vi "prototype-02.vi"() -> ()   [LabVIEW 2026]
uses:
  <vilib>/Instr/_visa.llb/VISA Configure Serial Port (Instr).vi
panel:
  in  "Numeric 3":dbl
  in  "Numeric 2":dbl
  in  "Numeric":dbl
  in  "TV":bool
  in  "BULB":bool
  in  "FAN":bool
  in  "VISA resource name":refnum<visa-resource-name>
  in  "stop":bool
  in  "Voltage":dbl(knob) scale=0.0..250.0
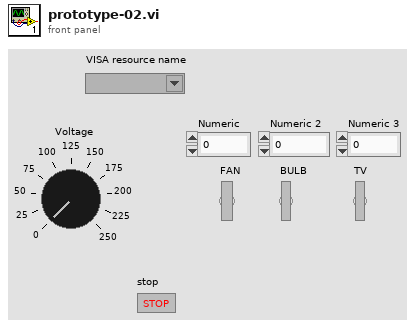
[diagram p1: front panel]
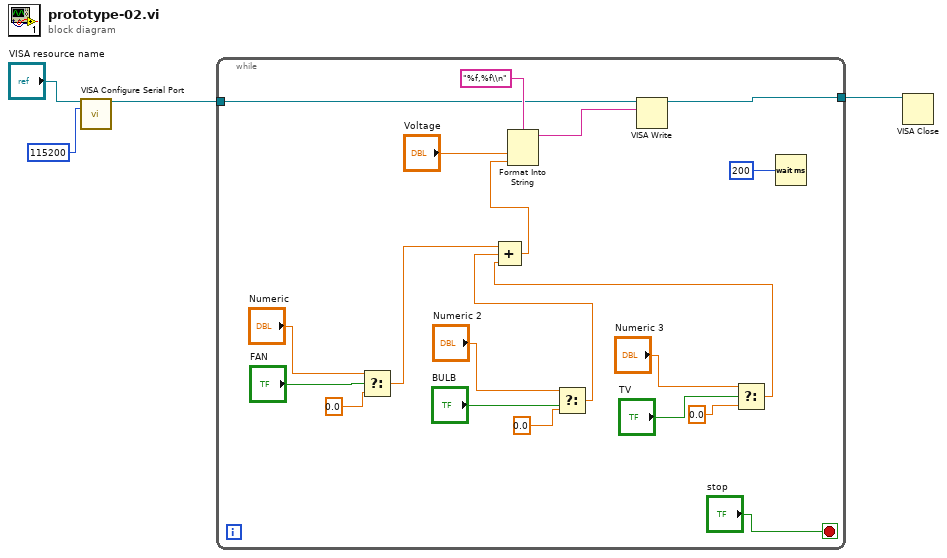
[diagram p0: block diagram]
diagram:
  n1 = call-poly "VISA Configure Serial Port"("VISA resource name"="VISA resource name", "baud rate (9600)"=u32 115200) -> ("VISA resource name out"=w2:refnum<visa-resource-name>)  [unwired: 12 in, 1 out]
  n2 = while {
    tunnel: w2 -> [w20]
    tunnel: [w19] -> w1
    stop <- "stop" stop-if-true
    n3 = Select(t="Numeric", s="FAN", f=0.0) -> (s? t:f=w16:dbl)
    n4 = Select(t="Numeric 2", s="BULB", f=0.0) -> (s? t:f=w8:dbl)
    n5 = Select(t="Numeric 3", s="TV", f=0.0) -> (s? t:f=w17:dbl)
    n6 = Compound Arithmetic op=ADD(w16, w8, w17) -> (w12:dbl)
    n7 = Format Into String "Format Into String"(format string="%f,%f\\n", "Voltage", w12) -> (resulting string=w21:string)  [unwired: 2 in, 1 out]
    n8 = VISA Write(VISA resource name=w20, write buffer=w21) -> (VISA resource name out=w19:refnum<visa-resource-name>)  [unwired: 1 in, 2 out]
    n9 = Wait (ms)(milliseconds to wait=u32 200) -> ()  [unwired: 1 out]
  }
  n10 = VISA Close(VISA resource name=w1) -> ()  [unwired: 1 in, 1 out]
